vi "Write BMP Data.vi"(4 "icon mask data":u8[](array[numeric]), 5 "bmp header":T1, 6 "data":u8[](array[numeric]), 7 "color table":u32[](array[colorbox]), 8 "error in (no error)":errorcluster, 9 "bmp is for icon? (F)":bool, 10 "offset":u32 format="%x", 11 "file path":refnum<file>) -> (0 "error out":errorcluster, 3 "file path copy":refnum<file>)   [LabVIEW 2020]
panel:
  in  "write\nCase Constant\n(See Context Help)":bool=TRUE
  out "?":string
  out "length":i32
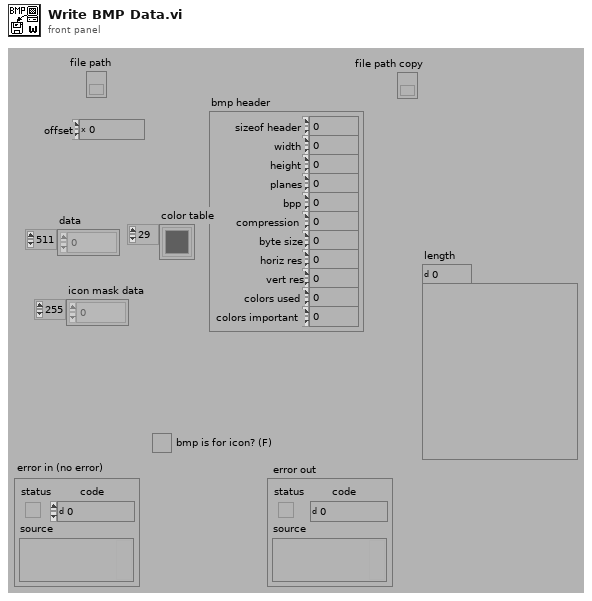
[diagram p1: front panel]
types:
  T1 = cluster{"sizeof header":u32, "width":u32, "height":u32, "planes":u16, "bpp":u16, "compression":u32, "byte size":u32, "horiz res":u32, "vert res":u32, "colors used":u32, "colors important":u32}
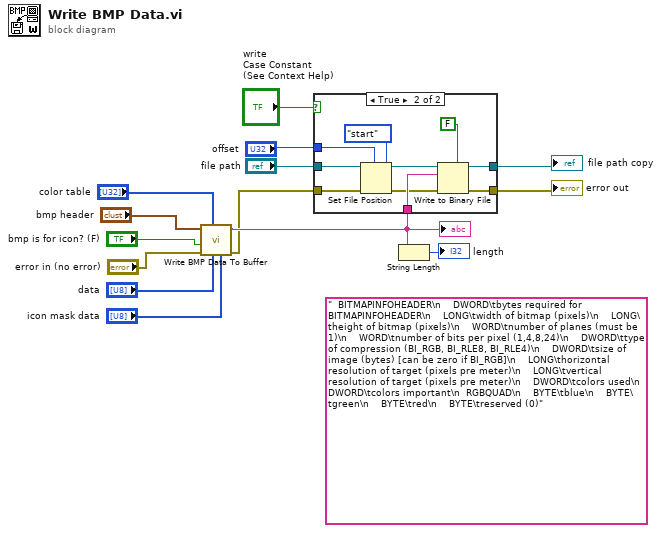
[diagram p0: block diagram]
diagram:
  (unwired) "  BITMAPINFOHEADER\n    DWORD\tbytes required for BITMAPINFOHEADER\n    LONG\twidth of bitmap (pixels)\n    LONG\theight of bitmap (pixels)\n    WORD\tnumber of planes (must be 1)\n    WORD\tnumber of bits per pixel (1,4,8,24)\n    DWORD\ttype of compression (BI_RGB, BI_RLE8, BI_RLE4)\n    DWORD\tsize of image (bytes) [can be zero if BI_RGB]\n    LONG\thorizontal resolution of target (pixels pre meter)\n    LONG\tvertical resolution of target (pixels pre meter)\n    DWORD\tcolors used\n    DWORD\tcolors important\n  RGBQUAD\n    BYTE\tblue\n    BYTE\tgreen\n    BYTE\tred\n    BYTE\treserved (0)"
  n1 = call "Write BMP Data To Buffer.vi"("icon mask data"="icon mask data", "data"="data", "color table"="color table", "error in (no error)"="error in (no error)", "bmp is for icon? (F)"="bmp is for icon? (F)", "bmp header"="bmp header") -> ("error out"=w5:errorcluster, "buffer"=w8:string)  [unwired: 4 in]
  "?" <- w8
  n2 = case shown="True" "write\nCase Constant\n(See Context Help)" {
    tunnel: w5 -> [w16 w26]
    tunnel: [w16 w25] -> w14
    tunnel: "file path" -> [w15 w24]
    tunnel: [w15 w23] -> w12
    tunnel: "offset" -> [_ w22]
    tunnel: w8 -> [_ w20]
    frame False {
    }
    frame True {
      n3 = Set File Position(offset (in bytes) (0)=w22, refnum=w24, from (0:start)=enum16{"start", "end", "current"}."start" ("pos mode (0:2)"), error in=w26) -> (refnum out=w19:refnum<file>, error out=w18:errorcluster)
      n4 = Write to Binary File(file (use dialog)=w19, data=w20, error in=w18, 5:FALSE ("prepend array or string size? (T)")) -> (refnum out=w23:refnum<file>, error out=w25:errorcluster)  [unwired: 2 in, 1 out]
    }
  }
  "file path copy" <- w12
  "error out" <- w14
  n5 = String Length(string=w8) -> (length=→"length":i32)
